vi "Get IVI Controls Name.vi"(11 "error in":errorcluster) -> (4 "control names out":string[](array[string]), 6 "array size":i32, 15 "error out":errorcluster)   [LabVIEW 2021, in "Converter Reusables.lvlib"]
uses:
  Converter Reusables.lvlib
  TypeDefs/Dictionary States.ctl
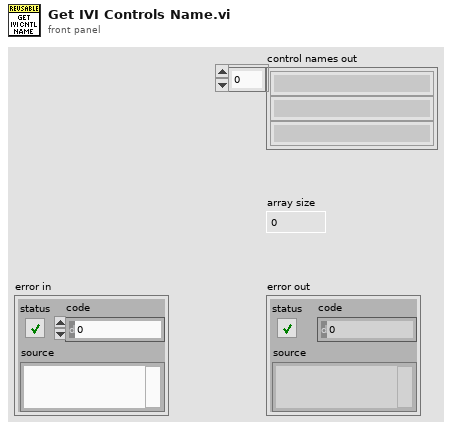
[diagram p1: front panel]
types:
  T1 = typedef "Converter Reusables.lvlib/Dictionary States.ctl" = enum16{"Set", "Get", "Delete", "Delete All"}
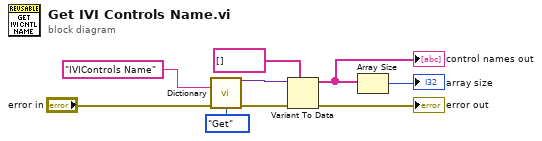
[diagram p0: block diagram]
diagram:
  n1 = call "Dictionary.vi"("key"="IVIControls Name" ("Key"), "error in"="error in", "dict states"=Dictionary_States."Get" ("Dict States")) -> ("variant out"=w5:variant, "error out"=w6:errorcluster)  [unwired: 11 in]
  n2 = Variant To Data(error in=w6, type=string[] [], Variant=w5) -> (data=w3:string[], error out=→"error out":errorcluster)
  "control names out" <- w3
  n3 = Array Size(array=w3) -> (size(s)=→"array size":i32)
